vi "Battery Switch States to Word.vi"(11 "Battery Switch States":T1) -> (3 "Battery Switch Word":u16)   [LabVIEW 2014, in "SLSC configuration Shared.lvlib"]
doc: "Converts four faults to a fault word."
uses:
  SLSC configuration Shared.lvlib
  Battery Switch Array.ctl
  Battery Switch.ctl
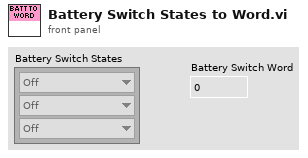
[diagram p1: front panel]
types:
  T1 = typedef "SLSC configuration Shared.lvlib/Battery Switch Array.ctl" = T2[]
  T2 = typedef "SLSC configuration Shared.lvlib/Battery Switch.ctl" = enum8{"Off", "On"}
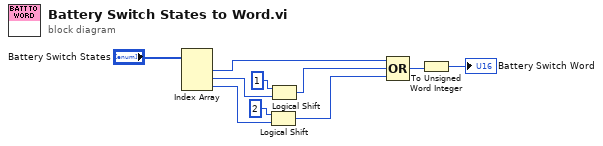
[diagram p0: block diagram]
diagram:
  n1 = Index Array(array="Battery Switch States") -> (element #1=w6:T2, element #2=w2:T2, element #3=w3:T2)  [unwired: 3 in]
  n2 = Logical Shift(y=u16 2, x=w3) -> (x << y=w8:u32)
  n3 = Logical Shift(y=u16 1, x=w2) -> (x << y=w7:u32)
  n4 = Compound Arithmetic op=OR(w6, w7, w8) -> (w9:u32)
  n5 = To Unsigned Word Integer(number=w9) -> (unsigned 16bit integer=→"Battery Switch Word":u16)
